vi "11.2.6.-Momentos Invariantes de Hu - Redes Neuronales.vi"() -> ()   [LabVIEW 2020]
panel:
  out "Figura Seleccionada (Pokemon):":string
  in  "Stop":bool
  out "Imagen Seleccionada":picture
  in  "Seleccionar imagen":bool
  # "Visión Artificial - Momentos Invariantes de Hu - Redes Neuronales\nDiego Cervantes Rodríguez\ndicer0.com"
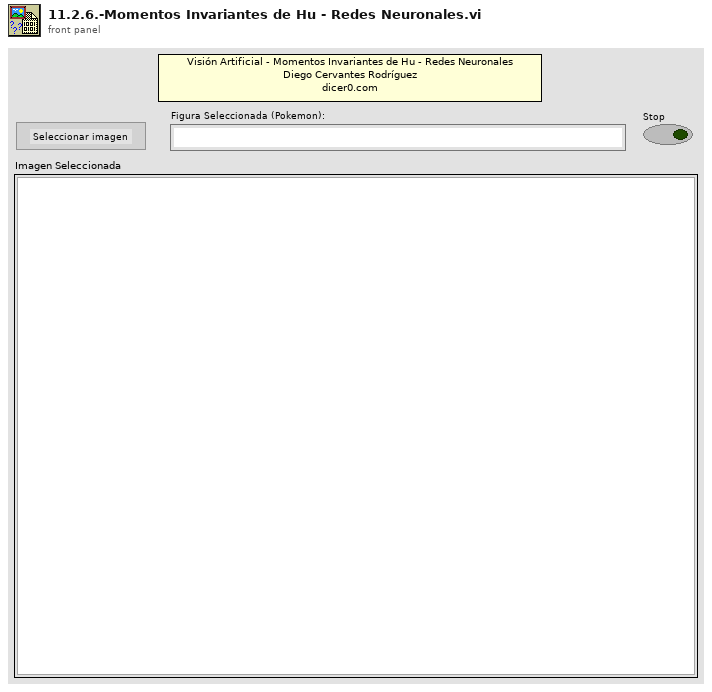
[diagram p1: front panel]
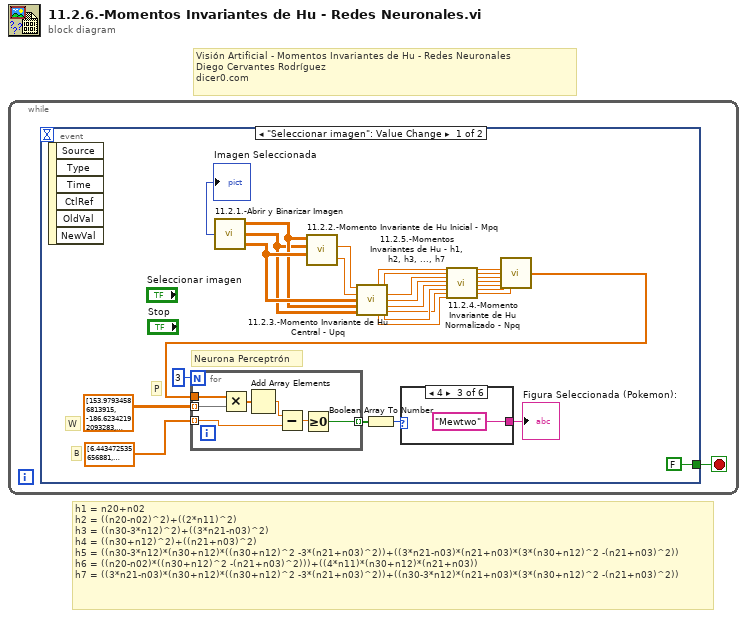
[diagram p0: block diagram]
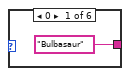
[diagram p2: hidden frame]
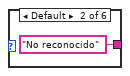
[diagram p3: hidden frame]
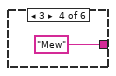
[diagram p4: hidden frame]
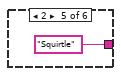
[diagram p5: hidden frame]
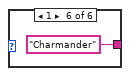
[diagram p6: hidden frame]
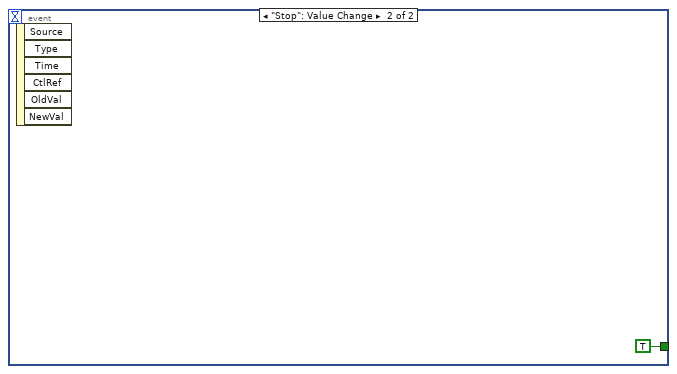
[diagram p7: hidden frame]
diagram:
  # "h1 = n20+n02\nh2 = ((n20-n02)^2)+((2*n11)^2)\nh3 = ((n30-3*n12)^2)+((3*n21-n03)^2)\nh4 = ((n30+n12)^2)+((n21+n03)^2)\nh5 = ((n30-3*n12)*(n30+n12)*((n30+n12)^2 -3*(n21+n03)^2))+((3*n21-n03)*(n21+n03)*(3*(n30+n12)^2 -(n21+n03)^2))\nh6 = ((n20-n02)*((n30+n12)^2 -(n21+n03)^2)))+((4*n11)*(n30+n12)*(n21+n03))\nh7 = ((3*n21-n03)*(n30+n12)*((n30+n12)^2 -3*(n21+n03)^2))+((n30-3*n12)*(n21+n03)*(3*(n30+n12)^2 -(n21+n03)^2))"
  # "Visión Artificial - Momentos Invariantes de Hu - Redes Neuronales\nDiego Cervantes Rodríguez\ndicer0.com"
  n1 = while {
    stop <- w1 stop-if-true
    # "PROGRAMA PRINCIPAL"
    n2 = event shown="[0] \"Seleccionar imagen\": Value Change" {
      selector: _ -> [_ _]
      dyn-events: _ -> [_ _]
      timeout: _ -> [_ _]
      tunnel: [FALSE TRUE] -> w1
      event "Seleccionar imagen": Value Change {
        # "Neurona Perceptrón"
        # "P"
        # "W"
        # "B"
        n3 = event-data() -> ()  [unwired: 1 in, 6 out]
        n4 = call "11.2.1.-Abrir y Binarizar Imagen.vi"() -> ("F"=w13:dbl[][], "Y"=w11:dbl[][], "X"=w12:dbl[][], "Imagen seleccionada"=→"Imagen Seleccionada":picture)  [unwired: 2 in]
        n5 = call "11.2.2.-Momento Invariante de Hu Inicial - Mpq.vi"("f"=w13, "Y"=w11, "X"=w12) -> ("xc"=w29:dbl, "yc"=w30:dbl)  [unwired: 4 in, 3 out]
        n6 = call "11.2.3.-Momento Invariante de Hu Central - Upq.vi"("xc"=w29, "yc"=w30, "f"=w13, "X"=w12, "Y"=w11) -> ("u00"=w28:dbl, "u11"=w27:dbl, "u12"=w26:dbl, "u02"=w25:dbl, "u20"=w24:dbl, "u30"=w18:dbl, "u03"=w17:dbl, "u21"=w23:dbl)  [unwired: 3 in]
        n7 = call "11.2.4.-Momento Invariante de Hu Normalizado - Npq.vi"("u00"=w28, "u11"=w27, "u12"=w26, "u02"=w25, "u20"=w24, "u21"=w23, "u03"=w17, "u30"=w18) -> ("n11"=w14:dbl, "n12"=w22:dbl, "n02"=w21:dbl, "n20"=w20:dbl, "n21"=w19:dbl, "n03"=w16:dbl, "n30"=w15:dbl)  [unwired: 13 in]
        n8 = call "11.2.5.-Momentos Invariantes de Hu - h1, h2, h3, ..., h7.vi"("n12"=w22, "n11"=w14, "n02"=w21, "n20"=w20, "n21"=w19, "n03"=w16, "n30"=w15) -> ("Momentos de Hu"=w6:dbl[])  [unwired: 8 in]
        n9 = for {
          N: 3 -> [_]
          tunnel: [w38] -> w8 mode=indexing
          tunnel: w6 -> [w40]
          tunnel: dbl[][] [[153.97934586813915, -186.62342192093283, -86.42595794341878, -58.234624680151214, -324.41429692489976, -148.83363301875147, 522.402755984038], [303.4838572643274, -337.6825976252579, -193.5313503864576, -10.257053966341353, 363.03172767953544, -6.360573614154783, -204.33838001357003], [-18.03575762869537, 175.4795424863235, 43.27558203410412, -45.75607617347369, -82.42105672322393, 36.91021644254077, -30.61701594675965]] ("w") -> [w37] mode=indexing
          tunnel: dbl[] [6.443472535656881, 6.064681563275089, 6.048871713080615] ("B") -> [w39] mode=indexing
          n10 = Multiply(x=w40, y=w37) -> (x*y=w42:dbl[])
          n11 = Add Array Elements(numeric array=w42) -> (sum=w41:dbl)
          n12 = Subtract(x=w41, y=w39) -> (x-y=w43:dbl)
          n13 = Greater Or Equal To 0?(x=w43) -> (x >= 0?=w38:bool)
        }
        n14 = Boolean Array To Number(Boolean array=w8) -> (number=w9:u32)
        n15 = case shown="4" w9 {
          tunnel: ["Bulbasaur" ("Personaje") "No reconocido" ("Personaje") "Mewtwo" ("Personaje") "Mew" ("Personaje") "Squirtle" ("Personaje") "Charmander" ("Personaje")] -> w5
          frame 0 {
          }
          frame Default {
          }
          frame 4 {
          }
          frame 3 {
          }
          frame 2 {
          }
          frame 1 {
          }
        }
        "Figura Seleccionada (Pokemon):" <- w5
      }
      event "Stop": Value Change {
        n16 = event-data() -> ()  [unwired: 1 in, 6 out]
      }
    }
  }
